vi "telemetria2.vi"(11 "Input can Array":string[][](array[string])) -> (0 "wiatr":T1 {"prêdkosc wiatru km/h" scale=0.0..50.0}, 1 "temp/wilg":T2, 2 "zap/kierunek":T3, 3 "wyj nowe P":cluster{"11":sgl, "12":sgl, "13":sgl}, 4 "output cluster":T4, 5 "wyj nowe L":cluster{"8":sgl, "9":sgl, "10":sgl}, 6 "ŒREDNIE NAPEDY":T7, 7 "MANIPULATOR wy":T5, 9 "pH":cluster{"temp. pkt rosy":sgl, "pH":sgl})   [LabVIEW 2015]
uses:
  <vilib>/ptbypt/NI_PtbyPt.lvlib
panel:
  out "wc 11":u16(graph)
  out "(hi.lo) 3":u16
  out "wc 10":u16(graph)
  out "(hi.lo) 2":u16
  out "wc 9":u16(graph)
  out "(hi.lo)":u16
  out "RAW NAPEDY":T6
  out "Prad Prawy":cluster{u16}(graph)
  out "Prad Lewy":cluster{i16}(graph)
  out "match + rest of string":string
  out "substring before match":string
  out "concatenated string":string
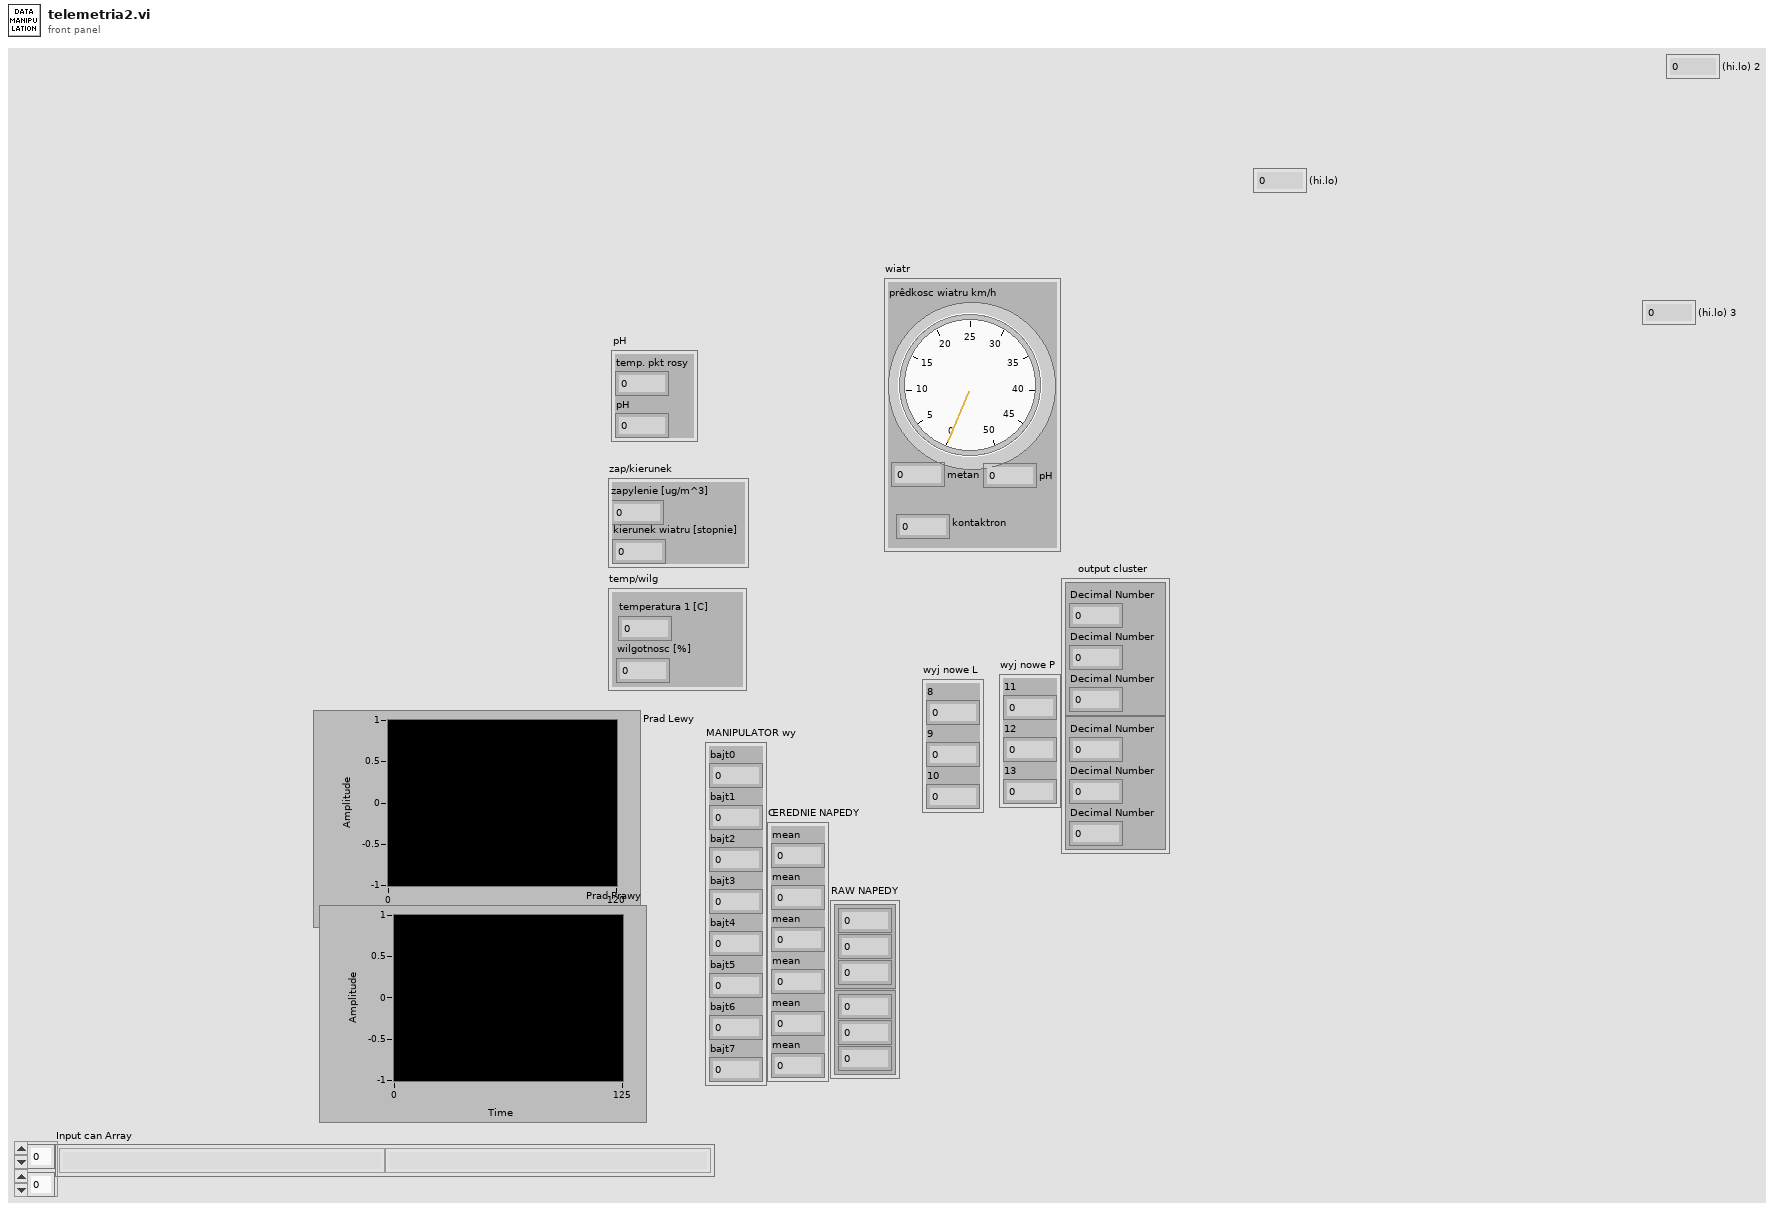
[diagram p1: front panel]
types:
  T1 = cluster{"pH":sgl, "metan":u8, "prêdkosc wiatru km/h":u16, "kontaktron":u8}
  T2 = cluster{"temperatura 1 [C]":sgl, "wilgotnosc [%]":sgl}
  T3 = cluster{"zapylenie [ug/m^3] ":sgl, "kierunek wiatru [stopnie]":sgl}
  T4 = cluster{cluster{"Decimal Number":sgl, "Decimal Number":sgl, "Decimal Number":sgl}, cluster{"Decimal Number":sgl, "Decimal Number":sgl, "Decimal Number":sgl}}
  T5 = cluster{"bajt0":u8, "bajt1":u16, "bajt2":u16, "bajt3":u16, "bajt4":u16, "bajt5":u16, "bajt6":u8, "bajt7":u8}
  T6 = cluster{cluster{i16, i16, i16}, cluster{i16, i16, i16}}
  T7 = cluster{"mean":dbl, "mean":dbl, "mean":dbl, "mean":dbl, "mean":dbl, "mean":dbl}
  T8 = cluster{"Decimal Number":sgl, "Decimal Number":sgl}
  T9 = cluster{"Decimal Number":sgl, "Decimal Number":sgl, "Decimal Number":sgl}
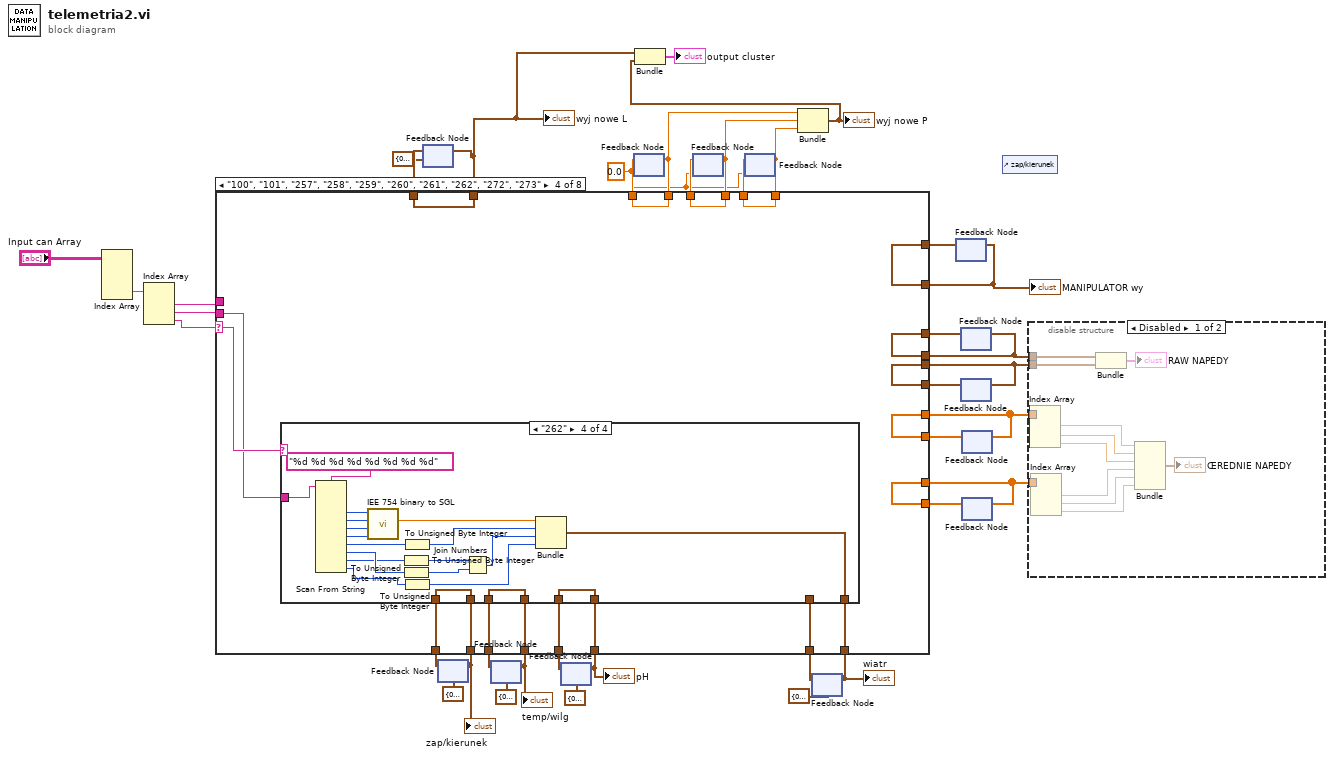
[diagram p0: block diagram]
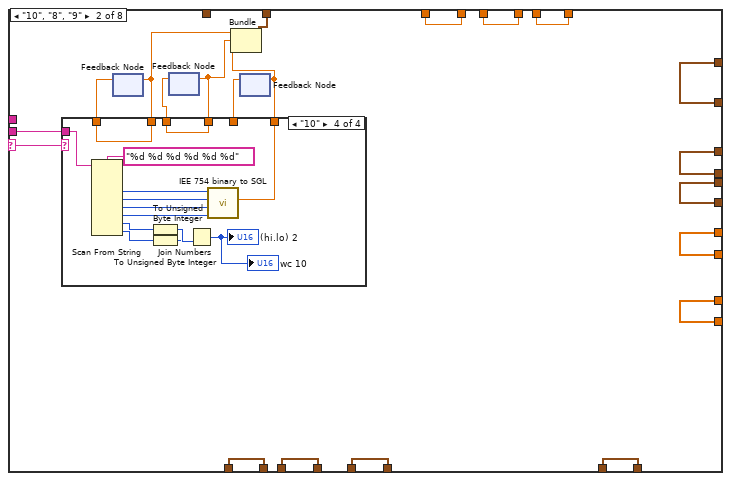
[diagram p4: hidden frame]
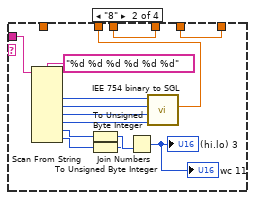
[diagram p6: hidden frame]
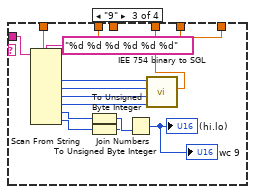
[diagram p7: hidden frame]
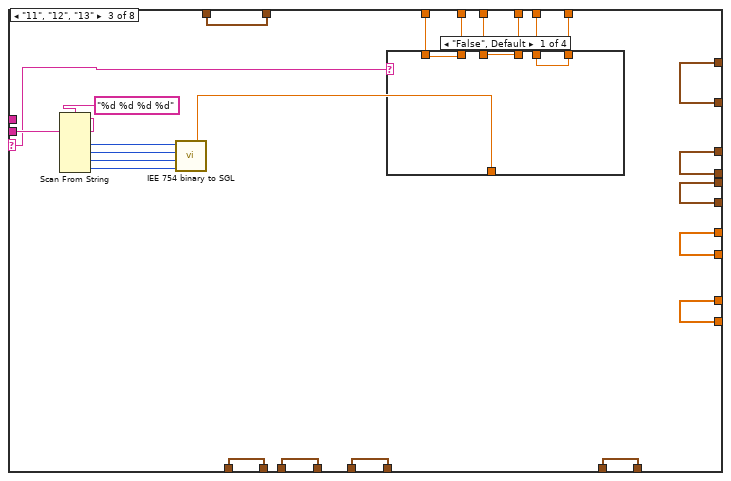
[diagram p8: hidden frame]
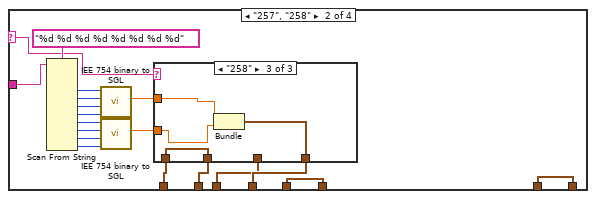
[diagram p13: hidden frame]
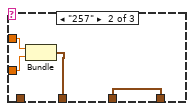
[diagram p15: hidden frame]
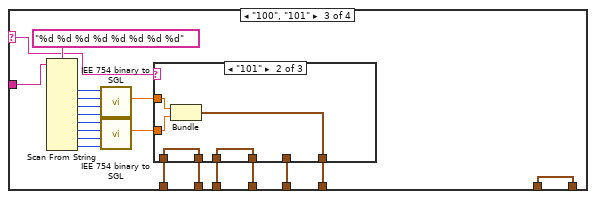
[diagram p16: hidden frame]
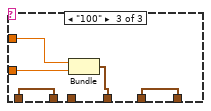
[diagram p18: hidden frame]
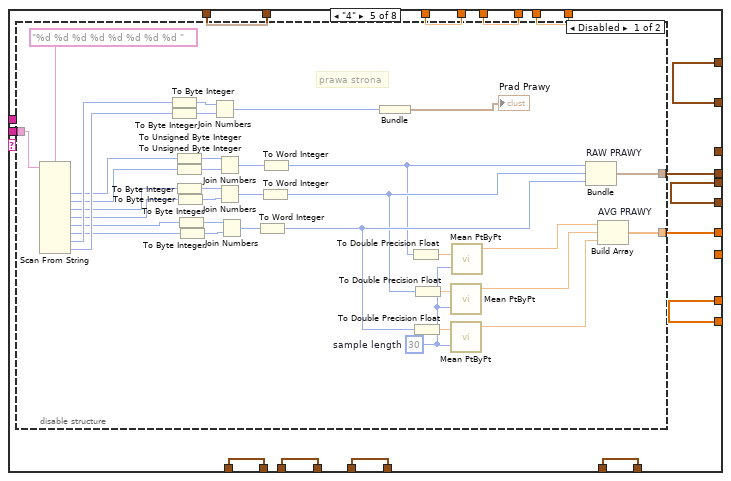
[diagram p19: hidden frame]
diagram:
  w8 = sgl 0.0 ("Decimal Number")
  n1 = Index Array(array="Input can Array") -> (element #2=w38:string[])  [unwired: 4 in, 1 out]
  n2 = Index Array(array=w38) -> (element #1=w35:string, element #2=w37:string, element #3=w25:string)  [unwired: 3 in]
  n3 = feedback #1(T9 {"Decimal Number"=0.0, "Decimal Number"=0.0, "Decimal Number"=0.0}) -> (w18:T9)
  n4 = feedback #2(T8 {"Decimal Number"=0.0, "Decimal Number"=0.0}) -> (w10:T8)
  n5 = feedback #3(T8 {"Decimal Number"=0.0, "Decimal Number"=0.0}) -> (w12:T8)
  n6 = feedback #4(T8 {"Decimal Number"=0.0, "Decimal Number"=0.0}) -> (w2:T8)
  n7 = feedback #5(w8) -> (w19:sgl)
  n8 = feedback #6(w8) -> (w20:sgl)
  n9 = feedback #7(w8) -> (w21:sgl)
  n10 = feedback #8(cluster{"Decimal Number":sgl, u8, u16, u8} {"Decimal Number"=0.0, 0, 0, 0}) -> (w14:cluster{"Decimal Number":sgl, u8, u16, u8})
  n11 = feedback #9() -> (w26:T5)  [unwired: 1 in]
  n12 = feedback #10() -> (w30:cluster{i16, i16, i16})  [unwired: 1 in]
  n13 = feedback #11() -> (w32:cluster{i16, i16, i16})  [unwired: 1 in]
  n14 = feedback #12() -> (w36:dbl[])  [unwired: 1 in]
  n15 = feedback #13() -> (w34:dbl[])  [unwired: 1 in]
  n16 = case shown="\"100\", \"101\", \"257\", \"258\", \"259\", \"260\", \"261\", \"262\", \"272\", \"273\"" w25 {
    selector: w25 -> [_ w68 w125 w170 _ _ _ _]
    tunnel: w37 -> [_ w57 w136 w163 w273 w322 w391 w414]
    tunnel: w36 -> [w49 w70 w139 w166 _ w319 w387 w403]
    tunnel: w35 -> [_ _ _ _ _ _ _ _]
    tunnel: [w52 w69 w138 w165 w272 w318 w390 w417] -> w28
    tunnel: w34 -> [w52 w69 w138 w165 w272 _ w390 w417]
    tunnel: [w50 w72 w141 w168 w271 w320 w388 w404] -> w31
    tunnel: [w51 w71 w140 w167 w270 w321 w389 w405] -> w33
    tunnel: w32 -> [w51 w71 w140 w167 w270 _ w389 w405]
    tunnel: w30 -> [w50 w72 w141 w168 _ w320 w388 w404]
    tunnel: [w49 w70 w139 w166 w269 w319 w387 w403] -> w29
    tunnel: [w48 w73 w142 w169 w268 w317 w377 w401] -> w27
    tunnel: w26 -> [w48 w73 w142 w169 w268 w317 _ w401]
    tunnel: [w47 w67 w126 w173 w267 w314 w363 w400] -> w22
    tunnel: w19 -> [w47 w67 w129 w173 w267 w314 w363 w400]
    tunnel: [w46 w66 w127 w172 w266 w315 w362 w399] -> w23
    tunnel: w20 -> [w46 w66 w130 w172 w266 w315 w362 w399]
    tunnel: [w45 w65 w128 w171 w265 w316 w361 w398] -> w24
    tunnel: w21 -> [w45 w65 w131 w171 w265 w316 w361 w398]
    tunnel: [w44 w60 w123 w164 w264 w313 w360 w397] -> w17
    tunnel: w18 -> [w44 _ w123 w164 w264 w313 w360 w397]
    tunnel: [w43 w56 w122 w162 w263 w312 w359 w396] -> w9
    tunnel: w14 -> [w43 w56 w122 w161 w263 w312 w359 w396]
    tunnel: [w42 w55 w121 w160 w262 w311 w358 w395] -> w13
    tunnel: w12 -> [w42 w55 w121 w159 w262 w311 w358 w395]
    tunnel: [w41 w54 w120 w158 w261 w310 w357 w394] -> w11
    tunnel: w10 -> [w41 w54 w120 w157 w261 w310 w357 w394]
    tunnel: [w40 w53 w119 w156 w260 w309 w356 w393] -> w3
    tunnel: w2 -> [w40 w53 w119 w155 w260 w309 w356 w393]
    frame "False", Default {
    }
    frame "10", "8", "9" {
      n17 = feedback #14() -> (w64:sgl)  [unwired: 1 in]
      n18 = feedback #15() -> (w58:sgl)  [unwired: 1 in]
      n19 = feedback #16() -> (w59:sgl)  [unwired: 1 in]
      n20 = case shown="\"10\"" w68 {
        tunnel: [w74 w77 w104 w118] -> w63
        tunnel: [w76 w90 w93 w117] -> w62
        tunnel: [w75 w89 w91 w105] -> w61
        tunnel: w64 -> [w74 _ w104 w118]
        tunnel: w59 -> [w75 w89 w91 _]
        tunnel: w58 -> [w76 w90 _ w117]
        tunnel: w57 -> [_ w78 w92 w106]
        frame "False", Default {
        }
        frame "8" {
          n21 = Scan From String(format string="%d %d %d %d %d %d", input string=w78) -> (output 1=w80:i32, output 2=w81:i32, output 3=w82:i32, output 4=w83:i32, output 5=w86:i32, output 6=w87:i32)  [unwired: 8 in, 3 out]
          n22 = To Unsigned Byte Integer(number=w86) -> (unsigned 8bit integer=w85:u8)
          n23 = To Unsigned Byte Integer(number=w87) -> (unsigned 8bit integer=w84:u8)
          n24 = Join Numbers(hi=w84, lo=w85) -> ((hi.lo)=→"(hi.lo) 3" →"wc 11":u16)
          n25 = call "IEE 754 binary to SGL.vi"("Numeric"=w83, "Numeric 2"=w82, "Numeric 3"=w81, "Numeric 4"=w80) -> ("Decimal Number"=w77:sgl)  [unwired: 7 in]
        }
        frame "9" {
          n26 = Scan From String(format string="%d %d %d %d %d %d", input string=w92) -> (output 1=w95:i32, output 2=w96:i32, output 3=w97:i32, output 4=w98:i32, output 5=w101:i32, output 6=w102:i32)  [unwired: 8 in, 3 out]
          n27 = To Unsigned Byte Integer(number=w101) -> (unsigned 8bit integer=w100:u8)
          n28 = To Unsigned Byte Integer(number=w102) -> (unsigned 8bit integer=w99:u8)
          n29 = Join Numbers(hi=w99, lo=w100) -> ((hi.lo)=→"(hi.lo)" →"wc 9":u16)
          n30 = call "IEE 754 binary to SGL.vi"("Numeric"=w98, "Numeric 2"=w97, "Numeric 3"=w96, "Numeric 4"=w95) -> ("Decimal Number"=w93:sgl)  [unwired: 7 in]
        }
        frame "10" {
          n31 = Scan From String(format string="%d %d %d %d %d %d", input string=w106) -> (output 1=w108:i32, output 2=w109:i32, output 3=w110:i32, output 4=w111:i32, output 5=w114:i32, output 6=w115:i32)  [unwired: 8 in, 3 out]
          n32 = To Unsigned Byte Integer(number=w114) -> (unsigned 8bit integer=w113:u8)
          n33 = To Unsigned Byte Integer(number=w115) -> (unsigned 8bit integer=w112:u8)
          n34 = Join Numbers(hi=w112, lo=w113) -> ((hi.lo)=→"(hi.lo) 2" →"wc 10":u16)
          n35 = call "IEE 754 binary to SGL.vi"("Numeric"=w111, "Numeric 2"=w110, "Numeric 3"=w109, "Numeric 4"=w108) -> ("Decimal Number"=w105:sgl)  [unwired: 7 in]
        }
      }
      n36 = feedback-in #14(w63) -> ()
      n37 = feedback-in #15(w62) -> ()
      n38 = Bundle("Decimal Number"=w63, "Decimal Number"=w62, "Decimal Number"=w61) -> (w60:T9)  [unwired: 1 in]
      n39 = feedback-in #16(w61) -> ()
    }
    frame "11", "12", "13" {
      n40 = Scan From String(format string="%d %d %d %d", input string=w136) -> (output 1=w135:i32, output 2=w134:i32, output 3=w133:i32, output 4=w132:i32)  [unwired: 6 in, 3 out]
      n41 = call "IEE 754 binary to SGL.vi"("Numeric"=w132, "Numeric 2"=w133, "Numeric 3"=w134, "Numeric 4"=w135) -> ("Decimal Number"=w124:sgl)  [unwired: 7 in]
      n42 = case shown="\"False\", Default" w125 {
        tunnel: [w145 w148 w150 w153] -> w126
        tunnel: w124 -> [_ w148 w151 w154]
        tunnel: [w144 w147 w151 w152] -> w127
        tunnel: [w143 w146 w149 w154] -> w128
        tunnel: w129 -> [w145 _ w150 w153]
        tunnel: w130 -> [w144 w147 _ w152]
        tunnel: w131 -> [w143 w146 w149 _]
        frame "False", Default {
        }
        frame "11" {
        }
        frame "12" {
        }
        frame "13" {
        }
      }
    }
    frame "100", "101", "257", "258", "259", "260", "261", "262", "272", "273" {
      n43 = case shown="\"262\"" w170 {
        selector: w170 -> [_ w184 w214 _]
        tunnel: w163 -> [_ w194 w224 w257]
        tunnel: [w177 w183 w213 w243] -> w162
        tunnel: w161 -> [w177 w183 w213 _]
        tunnel: [w176 w182 w212 w242] -> w160
        tunnel: w159 -> [w176 w181 w211 w242]
        tunnel: [w175 w180 w210 w241] -> w158
        tunnel: w157 -> [w175 w179 w209 w241]
        tunnel: [w174 w178 w208 w240] -> w156
        tunnel: w155 -> [w174 w178 w207 w240]
        frame "False", Default {
        }
        frame "257", "258" {
          n44 = Scan From String(format string="%d %d %d %d %d %d %d %d", input string=w194) -> (output 1=w193:i32, output 2=w192:i32, output 3=w190:i32, output 4=w189:i32, output 5=w188:i32, output 6=w187:i32, output 7=w186:i32, output 8=w185:i32)  [unwired: 10 in, 3 out]
          n45 = call "IEE 754 binary to SGL.vi"("Numeric"=w189, "Numeric 2"=w190, "Numeric 3"=w192, "Numeric 4"=w193) -> ("Decimal Number"=w196:sgl)  [unwired: 7 in]
          n46 = call "IEE 754 binary to SGL.vi"("Numeric"=w185, "Numeric 2"=w186, "Numeric 3"=w187, "Numeric 4"=w188) -> ("Decimal Number"=w195:sgl)  [unwired: 7 in]
          n47 = case shown="\"258\"" w184 {
            tunnel: w196 -> [_ w202 w206]
            tunnel: w195 -> [_ w201 w205]
            tunnel: [w198 w200 w204] -> w182
            tunnel: w181 -> [w198 w200 _]
            tunnel: [w197 w199 w203] -> w180
            tunnel: w179 -> [w197 _ w203]
            frame "False", Default {
            }
            frame "257" {
              n48 = Bundle("Decimal Number"=w202, "Decimal Number"=w201) -> (w199:T8)  [unwired: 1 in]
            }
            frame "258" {
              n49 = Bundle("Decimal Number"=w206, "Decimal Number"=w205) -> (w204:T8)  [unwired: 1 in]
            }
          }
        }
        frame "100", "101" {
          n50 = Scan From String(format string="%d %d %d %d %d %d %d %d", input string=w224) -> (output 1=w223:i32, output 2=w222:i32, output 3=w220:i32, output 4=w219:i32, output 5=w218:i32, output 6=w217:i32, output 7=w216:i32, output 8=w215:i32)  [unwired: 10 in, 3 out]
          n51 = call "IEE 754 binary to SGL.vi"("Numeric"=w219, "Numeric 2"=w220, "Numeric 3"=w222, "Numeric 4"=w223) -> ("Decimal Number"=w226:sgl)  [unwired: 7 in]
          n52 = call "IEE 754 binary to SGL.vi"("Numeric"=w215, "Numeric 2"=w216, "Numeric 3"=w217, "Numeric 4"=w218) -> ("Decimal Number"=w225:sgl)  [unwired: 7 in]
          n53 = case shown="\"101\"" w214 {
            tunnel: w226 -> [_ w234 w239]
            tunnel: w225 -> [_ w233 w238]
            tunnel: [w229 w232 w236] -> w212
            tunnel: w211 -> [w229 w232 _]
            tunnel: [w228 w231 w237] -> w210
            tunnel: w209 -> [w228 w231 w237]
            tunnel: [w227 w230 w235] -> w208
            tunnel: w207 -> [w227 _ w235]
            frame "False", Default {
            }
            frame "101" {
              n54 = Bundle("Decimal Number"=w234, "Decimal Number"=w233) -> (w230:T8)  [unwired: 1 in]
            }
            frame "100" {
              n55 = Bundle("Decimal Number"=w239, "Decimal Number"=w238) -> (w236:T8)  [unwired: 1 in]
            }
          }
        }
        frame "262" {
          n56 = Scan From String(format string="%d %d %d %d %d %d %d %d", input string=w257) -> (output 1=w252:i32, output 2=w251:i32, output 3=w250:i32, output 4=w249:i32, output 5=w253:i32, output 6=w255:i32, output 7=w254:i32, output 8=w248:i32)  [unwired: 10 in, 3 out]
          n57 = call "IEE 754 binary to SGL.vi"("Numeric"=w249, "Numeric 2"=w250, "Numeric 3"=w251, "Numeric 4"=w252) -> ("Decimal Number"=w247:sgl)  [unwired: 7 in]
          n58 = To Unsigned Byte Integer(number=w254) -> (unsigned 8bit integer=w259:u8)
          n59 = To Unsigned Byte Integer(number=w255) -> (unsigned 8bit integer=w258:u8)
          n60 = To Unsigned Byte Integer(number=w253) -> (unsigned 8bit integer=w246:u8)
          n61 = To Unsigned Byte Integer(number=w248) -> (unsigned 8bit integer=w244:u8)
          n62 = Join Numbers(hi=w259, lo=w258) -> ((hi.lo)=w245:u16)
          n63 = Bundle("Decimal Number"=w247, w246, w245, w244) -> (w243:cluster{"Decimal Number":sgl, u8, u16, u8})  [unwired: 1 in]
        }
      }
    }
    frame "4" {
      n64 = disable-structure shown="Disabled" {
        disable-tunnel: w273 -> [w307 _]
        disable-tunnel: [w299 _] -> w271
        disable-tunnel: [w295 _] -> w269
        frame Disabled {
          w282 = 30  # sample length
          # "prawa strona"
          n65 = Scan From String(format string="%d %d %d %d %d %d %d %d ", input string=w307) -> (output 1=w285:i32, output 2=w286:i32, output 3=w287:i32, output 4=w288:i32, output 5=w289:i32, output 6=w290:i32, output 7=w306:i32, output 8=w305:i32)  [unwired: 10 in, 3 out]
          n66 = To Byte Integer(number=w306) -> (8bit integer=w304:i8)
          n67 = To Byte Integer(number=w305) -> (8bit integer=w303:i8)
          n68 = To Unsigned Byte Integer(number=w285) -> (unsigned 8bit integer=w301:u8)
          n69 = To Unsigned Byte Integer(number=w286) -> (unsigned 8bit integer=w300:u8)
          n70 = To Byte Integer(number=w287) -> (8bit integer=w293:i8)
          n71 = To Byte Integer(number=w288) -> (8bit integer=w294:i8)
          n72 = To Byte Integer(number=w289) -> (8bit integer=w292:i8)
          n73 = To Byte Integer(number=w290) -> (8bit integer=w291:i8)
          n74 = Join Numbers(hi=w304, lo=w303) -> ((hi.lo)=w302:u16)
          n75 = Join Numbers(hi=w301, lo=w300) -> ((hi.lo)=w284:u16)
          n76 = Join Numbers(hi=w293, lo=w294) -> ((hi.lo)=w283:u16)
          n77 = Join Numbers(hi=w292, lo=w291) -> ((hi.lo)=w278:u16)
          n78 = To Word Integer(number=w278) -> (16bit integer=w277:i16)
          n79 = To Word Integer(number=w283) -> (16bit integer=w276:i16)
          n80 = To Word Integer(number=w284) -> (16bit integer=w275:i16)
          n81 = Bundle(w302) -> (→"Prad Prawy":cluster{u16})  [unwired: 1 in]
          n82 = To Double Precision Float(number=w275) -> (double precision float=w281:dbl)
          n83 = To Double Precision Float(number=w277) -> (double precision float=w279:dbl)
          n84 = To Double Precision Float(number=w276) -> (double precision float=w280:dbl)
          n85 = call <vilib>:"Mean PtByPt.vi"("x"=w280, "sample length"=w282) -> ("mean"=w297:dbl)  [unwired: 2 in, 1 out]
          n86 = call <vilib>:"Mean PtByPt.vi"("x"=w279, "sample length"=w282) -> ("mean"=w296:dbl)  [unwired: 2 in, 1 out]
          n87 = call <vilib>:"Mean PtByPt.vi"("x"=w281, "sample length"=w282) -> ("mean"=w298:dbl)  [unwired: 2 in, 1 out]
          n88 = Bundle "RAW PRAWY"(w275, w276, w277) -> (w299:cluster{i16, i16, i16})  [unwired: 1 in]
          n89 = Build Array "AVG PRAWY"(w298, w297, w296) -> (w295:dbl[])
        }
        frame Enabled {
        }
      }
    }
    frame "5" {
      n90 = disable-structure shown="Disabled" {
        disable-tunnel: w322 -> [w354 _]
        disable-tunnel: [w349 _] -> w321
        disable-tunnel: [w345 _] -> w318
        frame Disabled {
          w326 = 30  # sample length
          # "lewa strona"
          n91 = Scan From String(format string="%d %d %d %d %d %d %d %d  ", input string=w354) -> (output 1=w341:i32, output 2=w340:i32, output 3=w335:i32, output 4=w337:i32, output 5=w334:i32, output 6=w333:i32, output 7=w352:i32, output 8=w350:i32)  [unwired: 10 in, 3 out]
          n92 = To Byte Integer(number=w335) -> (8bit integer=w339:i8)
          n93 = To Byte Integer(number=w337) -> (8bit integer=w338:i8)
          n94 = To Byte Integer(number=w334) -> (8bit integer=w332:i8)
          n95 = To Byte Integer(number=w333) -> (8bit integer=w331:i8)
          n96 = To Byte Integer(number=w341) -> (8bit integer=w336:i8)
          n97 = To Byte Integer(number=w340) -> (8bit integer=w342:i8)
          n98 = Join Numbers(hi=w339, lo=w338) -> ((hi.lo)=w327:u16)
          n99 = Join Numbers(hi=w336, lo=w342) -> ((hi.lo)=w330:u16)
          n100 = Join Numbers(hi=w332, lo=w331) -> ((hi.lo)=w328:u16)
          n101 = To Word Integer(number=w328) -> (16bit integer=w324:i16)
          n102 = To Word Integer(number=w330) -> (16bit integer=w329:i16)
          n103 = To Word Integer(number=w327) -> (16bit integer=w325:i16)
          n104 = To Byte Integer(number=w352) -> (8bit integer=w353:i8)
          n105 = To Byte Integer(number=w350) -> (8bit integer=w351:i8)
          n106 = Join Numbers(hi=w353, lo=w351) -> ((hi.lo)=w343:u16)
          n107 = To Word Integer(number=w343) -> (16bit integer=w344:i16)
          n108 = Bundle(w344) -> (→"Prad Lewy":cluster{i16})  [unwired: 1 in]
          n109 = call <vilib>:"Mean PtByPt.vi"("x"=w329, "sample length"=w326) -> ("mean"=w348:dbl)  [unwired: 2 in, 1 out]
          n110 = call <vilib>:"Mean PtByPt.vi"("x"=w325, "sample length"=w326) -> ("mean"=w347:dbl)  [unwired: 2 in, 1 out]
          n111 = call <vilib>:"Mean PtByPt.vi"("x"=w324, "sample length"=w326) -> ("mean"=w346:dbl)  [unwired: 2 in, 1 out]
          n112 = Bundle ("RAW LEWY")(w329, w325, w324) -> (w349:cluster{i16, i16, i16})  [unwired: 1 in]
          n113 = Build Array "AVG LEWY"(w348, w347, w346) -> (w345:dbl[])
        }
        frame Enabled {
        }
      }
    }
    frame "32" {
      # "manipulator"
      n114 = Scan From String(format string="%d %d %d %d %d %d %d %d ", input string=w391) -> (output 1=w386:i32, output 2=w385:i32, output 3=w384:i32, output 4=w383:i32, output 5=w382:i32, output 6=w381:i32, output 7=w380:i32, output 8=w379:i32)  [unwired: 10 in, 3 out]
      n115 = To Unsigned Byte Integer(number=w386) -> (unsigned 8bit integer=w376:u8)
      n116 = To Unsigned Byte Integer(number=w385) -> (unsigned 8bit integer=w375:u8)
      n117 = To Unsigned Byte Integer(number=w384) -> (unsigned 8bit integer=w374:u8)
      n118 = To Unsigned Byte Integer(number=w383) -> (unsigned 8bit integer=w373:u8)
      n119 = To Unsigned Byte Integer(number=w382) -> (unsigned 8bit integer=w371:u8)
      n120 = To Unsigned Byte Integer(number=w381) -> (unsigned 8bit integer=w369:u8)
      n121 = To Unsigned Byte Integer(number=w380) -> (unsigned 8bit integer=w372:u8)
      n122 = To Unsigned Byte Integer(number=w379) -> (unsigned 8bit integer=w370:u8)
      n123 = call "skladanie bitow manipulator.vi"("bajt 3 in"=w373, "bajt 4 in"=w371, "bajt 5 in"=w369, "bajt 6 in"=w372, "bajt 2 in"=w374, "bajt 7 in"=w370, "bajt 1 in"=w375) -> ("bajt 1"=w368:u16, "bajt 2"=w367:u16, "bajt 3"=w366:u16, "babjt 4"=w365:u16, "bajt 5"=w364:u16)  [unwired: 16 in]
      n124 = Bundle By Name(cluster=T5 {"bajt0"=0, "bajt1"=0, "bajt2"=0, "bajt3"=0, "bajt4"=0, "bajt5"=0, "bajt6"=0, "bajt7"=0} ("MANIPULATOR can"), "bajt0"=w376, "bajt1"=w368, "bajt2"=w367, "bajt3"=w366, "bajt4"=w365, "bajt5"=w364, "bajt6"=w372, "bajt7"=w370) -> (w377:T5)
    }
    frame "      1100" {
      n125 = String Subset(string=w414, length (rest)=31 ("length (rest)")) -> (substring=w412:string)  [unwired: 1 in]
      n126 = Spreadsheet String To Array(format string="%s", spreadsheet string=w412, array type (2D Dbl)=u8[] [] ("unsigned byte array")) -> (array=w411:u8[])  [unwired: 1 in]
      n127 = Byte Array To String(unsigned byte array=w411) -> (string=w406:string)
      n128 = feedback #17() -> (w410:string)  [unwired: 1 in]
      "concatenated string" <- w410
      n129 = Concatenate Strings(w406, w410) -> (w409:string)
      n130 = feedback-in #17(w409) -> ()
      n131 = Search/Split String(string=w409, search string/char (-)="#") -> (substring before match=→"substring before match":string, match + rest of string=→"match + rest of string":string)  [unwired: 1 in, 1 out]
    }
  }
  "wyj nowe L" <- w17
  "MANIPULATOR wy" <- w27
  "temp/wilg" <- w13
  "zap/kierunek" <- w11
  "wiatr" <- w9
  "pH" <- w3
  n132 = feedback-in #1(w17) -> ()
  n133 = feedback-in #2(w11) -> ()
  n134 = feedback-in #3(w13) -> ()
  n135 = feedback-in #4(w3) -> ()
  n136 = feedback-in #5(w22) -> ()
  n137 = feedback-in #6(w23) -> ()
  n138 = feedback-in #7(w24) -> ()
  n139 = Bundle("Decimal Number"=w22, "Decimal Number"=w23, "Decimal Number"=w24) -> (w16:T9)  [unwired: 1 in]
  "wyj nowe P" <- w16
  n140 = Bundle(w17, w16) -> (→"output cluster":T4)  [unwired: 1 in]
  n141 = feedback-in #8(w9) -> ()
  n142 = feedback-in #9(w27) -> ()
  n143 = feedback-in #10(w31) -> ()
  n144 = feedback-in #11(w33) -> ()
  n145 = feedback-in #12(w29) -> ()
  n146 = feedback-in #13(w28) -> ()
  n147 = control-ref of="zap/kierunek"() -> ()  [unwired: 1 out]
  n148 = disable-structure shown="Disabled" {
    disable-tunnel: w33 -> [w429 _]
    disable-tunnel: w31 -> [w428 _]
    disable-tunnel: w29 -> [w427 _]
    disable-tunnel: w28 -> [w426 _]
    frame Disabled {
      n149 = Index Array(array=w427) -> (element #1=w424:dbl, element #2=w423:dbl, element #3=w422:dbl)  [unwired: 3 in]
      n150 = Index Array(array=w426) -> (element #1=w421:dbl, element #2=w420:dbl, element #3=w419:dbl)  [unwired: 3 in]
      n151 = Bundle ("RAW NAPEDY")(w428, w429) -> (→"RAW NAPEDY":T6)  [unwired: 1 in]
      n152 = Bundle("mean"=w424, "mean"=w423, "mean"=w422, "mean"=w421, "mean"=w420, "mean"=w419) -> (→"ŒREDNIE NAPEDY":T7)  [unwired: 1 in]
    }
    frame Enabled {
    }
  }
